vi "骰子比大小.vi"() -> ()   [LabVIEW 2014]
panel:
  in  "Listbox 3":i32[](listbox)
  in  "Listbox 2":i32[](listbox)
  in  "Listbox":i32[](listbox)
  in  "遊戲開始":bool
  out "賺取/賠掉金額總計":i32
  out "歷經輪數":i32
  out "此輪賺取/賠掉金額":i32
  out "賭金金額":i32
  in  "Cluster 12":T1={"Color Box 4"=16448250, "Boolean 5"=FALSE, "Boolean 11"=FALSE, "Boolean 12"=FALSE, "Boolean 13"=FALSE, "Boolean 14"=FALSE, "Boolean 15"=FALSE}
  in  "Cluster 11":T2={"Color Box"=16777215, "Boolean 4"=FALSE, "Boolean 5"=FALSE, "Boolean 6"=FALSE, "Boolean 7"=FALSE, "Boolean 8"=FALSE}
  in  "Cluster 10":T3={"Color Box 2"=16777215, "Boolean 3"=FALSE, "Boolean 4"=FALSE, "Boolean 6"=FALSE, "Boolean 5"=FALSE}
  in  "Cluster 9":T4={"Color Box 2"=16777215, "Boolean"=FALSE, "Boolean 3"=FALSE, "Boolean 2"=FALSE}
  in  "Cluster 8":T5={"Color Box"=16777215, "Boolean"=FALSE, "Boolean 2"=FALSE}
  in  "Cluster 7":T6={"Color Box"=16777215, "Boolean"=FALSE}
  in  "Cluster 6":T1={"Color Box 4"=16448250, "Boolean 5"=FALSE, "Boolean 11"=FALSE, "Boolean 12"=FALSE, "Boolean 13"=FALSE, "Boolean 14"=FALSE, "Boolean 15"=FALSE}
  in  "Cluster 5":T2={"Color Box"=16777215, "Boolean 4"=FALSE, "Boolean 5"=FALSE, "Boolean 6"=FALSE, "Boolean 7"=FALSE, "Boolean 8"=FALSE}
  in  "Cluster 4":T3={"Color Box 2"=16777215, "Boolean 3"=FALSE, "Boolean 4"=FALSE, "Boolean 6"=FALSE, "Boolean 5"=FALSE}
  in  "Cluster 3":T4={"Color Box 2"=16777215, "Boolean"=FALSE, "Boolean 3"=FALSE, "Boolean 2"=FALSE}
  in  "Cluster 2":T5={"Color Box"=16777215, "Boolean"=FALSE, "Boolean 2"=FALSE}
  in  "Cluster":T6={"Color Box"=16777215, "Boolean"=FALSE}
  in  "下注金額":i32=10 min=10 max=30
  in  "賠率":i32=1 min=1 max=5
  in  "進入下一輪":bool
  in  "停止擲骰子":bool
  in  "退出遊戲":bool
  out "莊家骰子點數":i32
  out "玩家骰子點數":i32
  # "遊戲介紹:"
  # "遊戲操作:"
  # "注意事項:"
  # "看完以上說明都沒問題的話，\n就可以按下遊戲開始開始遊玩囉!\n                         ↓"
  # "莊家骰子點數"
  # "玩家骰子點數"
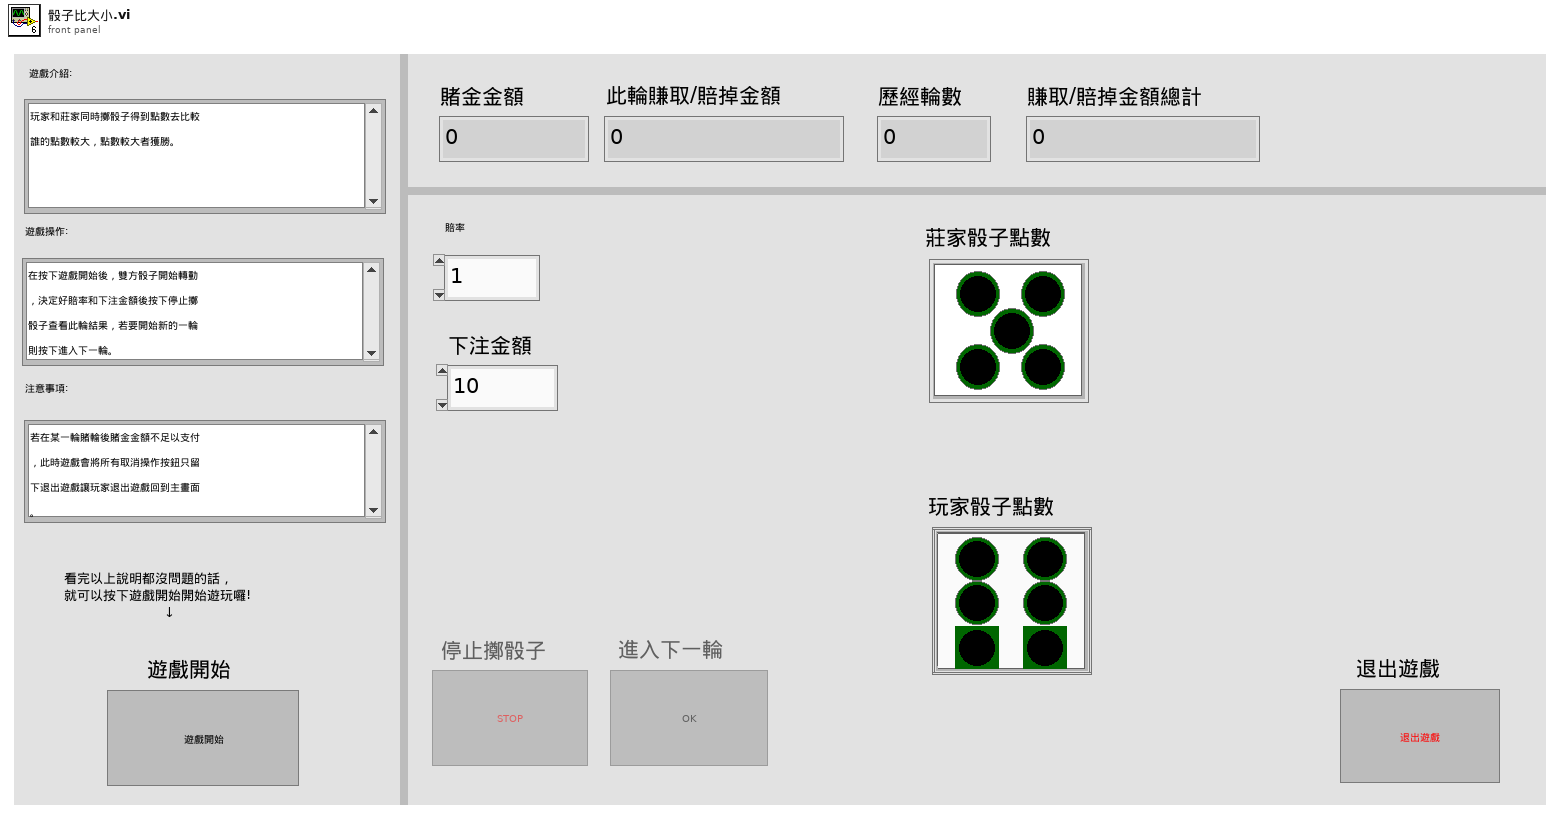
[diagram p1: front panel]
types:
  T1 = typedef "點數六.ctl" = cluster{"Color Box 4":u32, "Boolean 5":bool, "Boolean 11":bool, "Boolean 12":bool, "Boolean 13":bool, "Boolean 14":bool, "Boolean 15":bool}
  T2 = typedef "き.ctl" = cluster{"Color Box":u32, "Boolean 4":bool, "Boolean 5":bool, "Boolean 6":bool, "Boolean 7":bool, "Boolean 8":bool}
  T3 = typedef "點數四.ctl" = cluster{"Color Box 2":u32, "Boolean 3":bool, "Boolean 4":bool, "Boolean 6":bool, "Boolean 5":bool}
  T4 = typedef "點數三.ctl" = cluster{"Color Box 2":u32, "Boolean":bool, "Boolean 3":bool, "Boolean 2":bool}
  T5 = typedef "點數二.ctl" = cluster{"Color Box":u32, "Boolean":bool, "Boolean 2":bool}
  T6 = typedef "點數一.ctl" = cluster{"Color Box":u32, "Boolean":bool}
  T7 = enum16{"restart", "wait start button press", "compare", "throw dice", "init"}
  T8 = enum8{"Enabled", "Disabled", "Disabled and Grayed Out"}
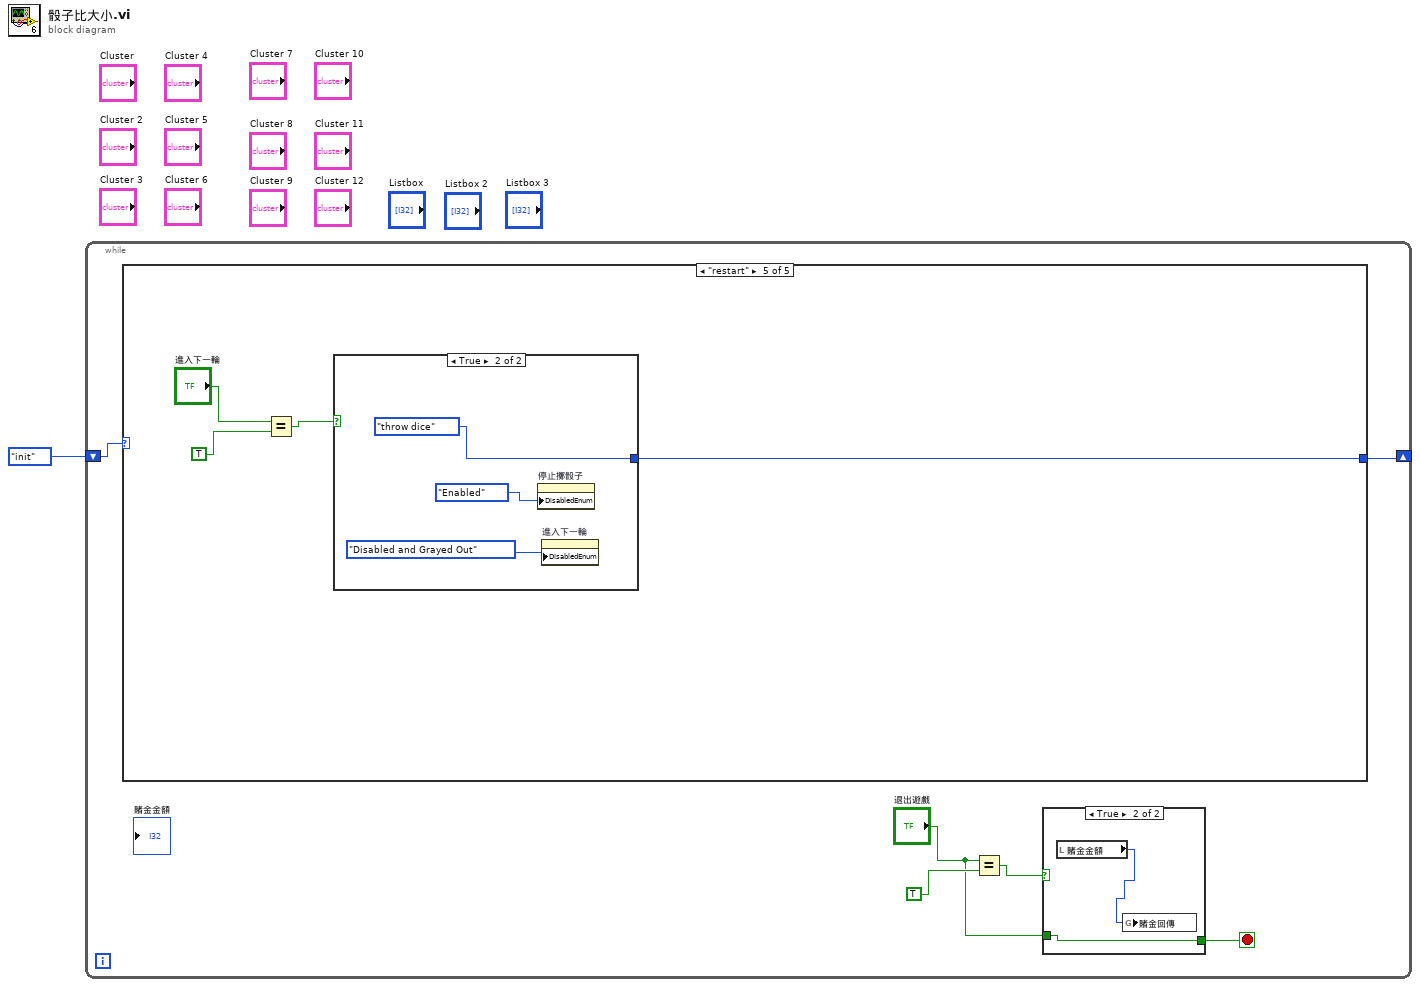
[diagram p0: block diagram]
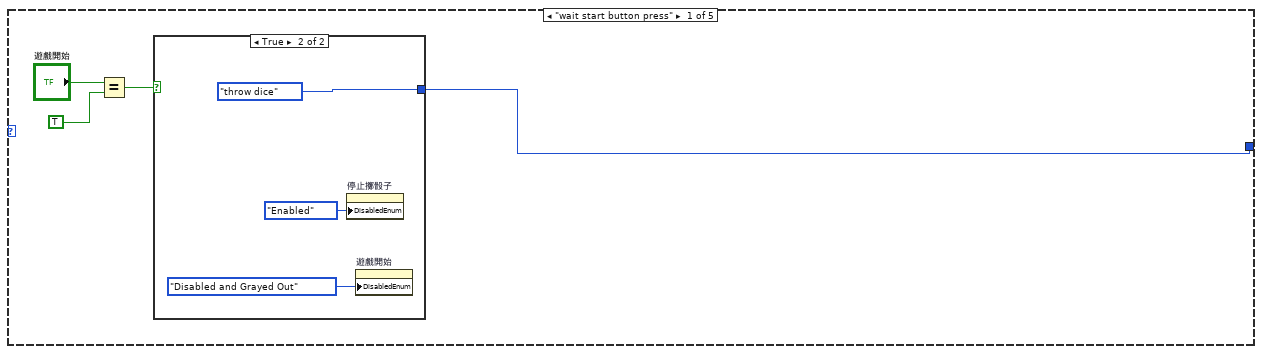
[diagram p3: hidden frame]
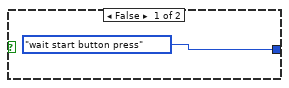
[diagram p4: hidden frame]
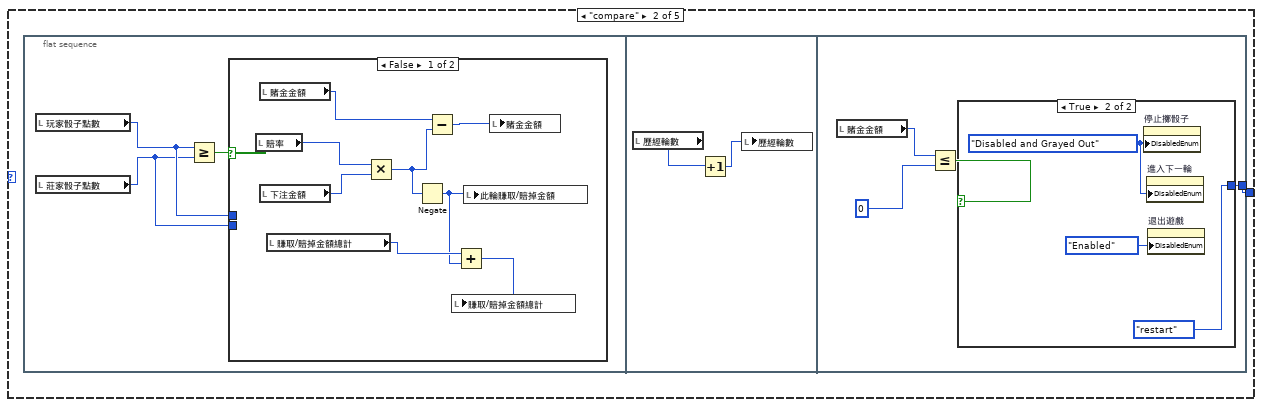
[diagram p5: hidden frame]
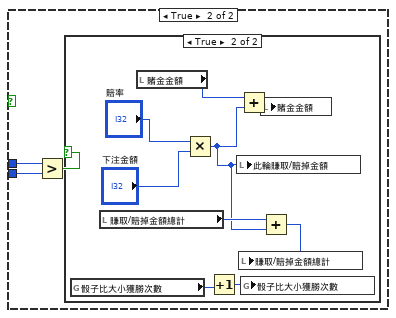
[diagram p6: hidden frame]
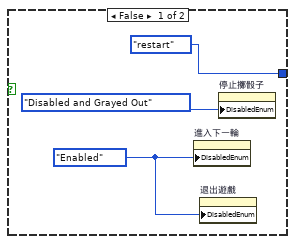
[diagram p8: hidden frame]
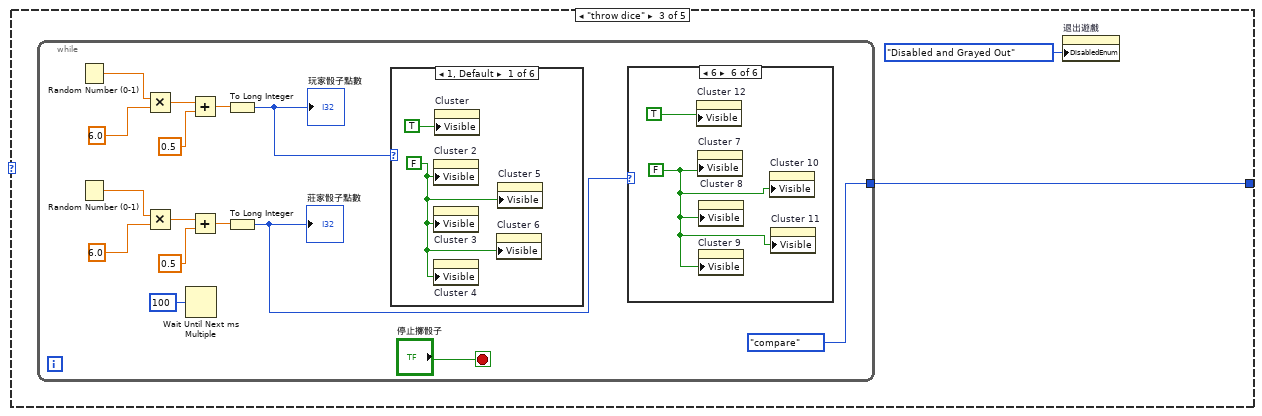
[diagram p9: hidden frame]
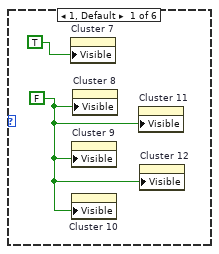
[diagram p10: hidden frame]
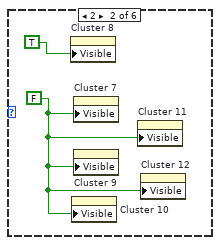
[diagram p11: hidden frame]
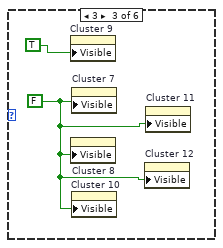
[diagram p12: hidden frame]
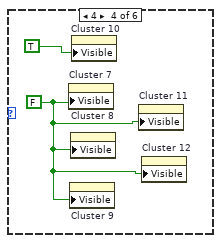
[diagram p13: hidden frame]
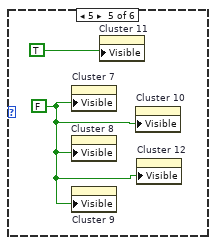
[diagram p14: hidden frame]
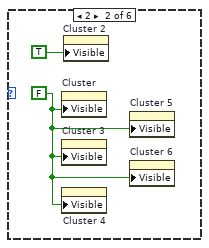
[diagram p15: hidden frame]
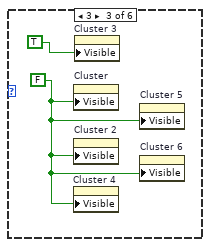
[diagram p16: hidden frame]
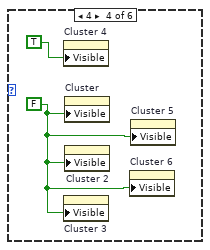
[diagram p17: hidden frame]
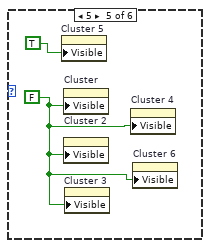
[diagram p18: hidden frame]
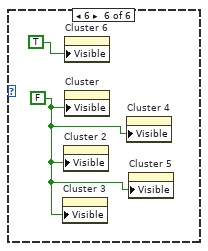
[diagram p19: hidden frame]
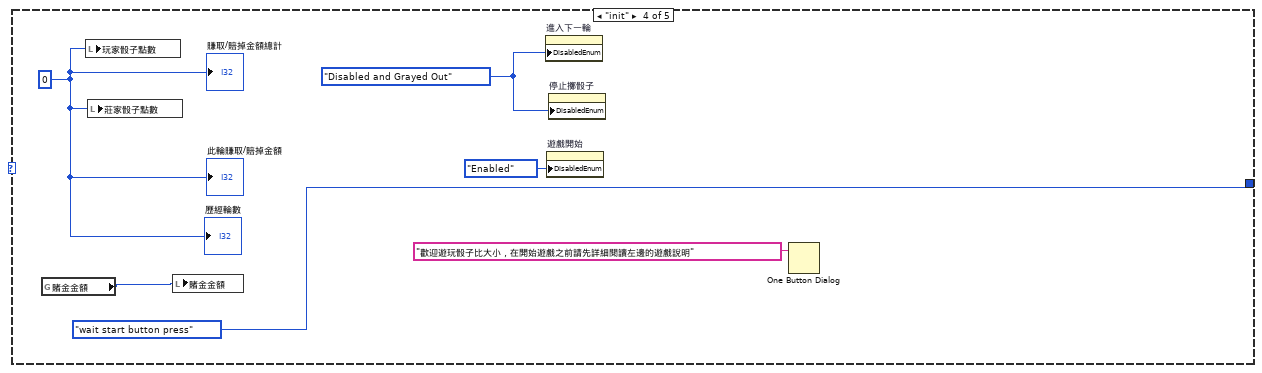
[diagram p20: hidden frame]
diagram:
  n1 = while {
    shift-right: [w6] -> _
    shift-left: T7."init" -> [w7]
    stop <- w3 stop-if-true
    n2 = case shown="\"restart\"" w7 {
      tunnel: [w11 w19 w56 T7."wait start button press" w102] -> w6
      frame "wait start button press" {
        n3 = Equal?(x="遊戲開始", y=TRUE) -> (x = y?=w12:bool)
        n4 = case shown="True" w12 {
          tunnel: [T7."wait start button press" T7."throw dice"] -> w11
          frame False {
          }
          frame True {
            n5 = property on="停止擲骰子" class="Bool"("DisabledEnum"=T8."Enabled" ("Disabled")) -> ()  [unwired: 2 in, 2 out]
            n6 = property on="遊戲開始" class="Bool (strict)"("DisabledEnum"=T8."Disabled and Grayed Out" ("Disabled")) -> ()  [unwired: 2 in, 2 out]
          }
        }
      }
      frame "compare" {
        n7 = flat-sequence {
          tunnel: [w45] -> w19
          frame #0 {
            n8 = local read "玩家骰子點數"() -> (w21:i32)
            n9 = local read "莊家骰子點數"() -> (w20:i32)
            n10 = Greater Or Equal?(x=w21, y=w20) -> (x >= y?=w22:bool)
            n11 = case shown="False" w22 {
              tunnel: w21 -> [_ w33]
              tunnel: w20 -> [_ w32]
              frame False {
                n12 = local read "賠率"() -> (w30:i32)
                n13 = local read "賭金金額"() -> (w28:i32)
                n14 = local read "下注金額"() -> (w29:i32)
                n15 = local read "賺取/賠掉金額總計"() -> (w25:i32)
                n16 = Multiply(x=w30, y=w29) -> (x*y=w26:i32)
                n17 = Negate(x=w26) -> (-x=w24:i32)
                n18 = Subtract(x=w28, y=w26) -> (x-y=w27:i32)
                n19 = Add(x=w25, y=w24) -> (x+y=w23:i32)
                n20 = local write "賺取/賠掉金額總計"(w23) -> ()
                n21 = local write "此輪賺取/賠掉金額"(w24) -> ()
                n22 = local write "賭金金額"(w27) -> ()
              }
              frame True {
                n23 = Greater?(x=w33, y=w32) -> (0:w31:bool)
                n24 = case shown="True" w31 {
                  frame False {
                  }
                  frame True {
                    n25 = global read "global variable-骰子比大小獲勝次數.vi" "骰子比大小獲勝次數"() -> (w34:i32)
                    n26 = local read "賺取/賠掉金額總計"() -> (w38:i32)
                    n27 = local read "賭金金額"() -> (w40:i32)
                    n28 = Multiply(x="賠率", y="下注金額") -> (x*y=w37:i32)
                    n29 = Increment(x=w34) -> (x+1=w35:i32)
                    n30 = local write "此輪賺取/賠掉金額"(w37) -> ()
                    n31 = Add(x=w40, y=w37) -> (x+y=w39:i32)
                    n32 = global write "global variable-骰子比大小獲勝次數.vi" "骰子比大小獲勝次數"(w35) -> ()
                    n33 = local write "賭金金額"(w39) -> ()
                    n34 = Add(x=w38, y=w37) -> (x+y=w36:i32)
                    n35 = local write "賺取/賠掉金額總計"(w36) -> ()
                  }
                }
              }
            }
          }
          frame #1 {
            n36 = local read "歷經輪數"() -> (w44:i32)
            n37 = Increment(x=w44) -> (x+1=w43:i32)
            n38 = local write "歷經輪數"(w43) -> ()
          }
          frame #2 {
            n39 = local read "賭金金額"() -> (w48:i32)
            n40 = Less Or Equal?(x=w48, y=0) -> (x <= y?=w46:bool)
            n41 = case shown="True" w46 {
              tunnel: [T7."restart" T7."restart"] -> w45
              frame False {
                w49 = T8."Enabled" ("Disabled")
                n42 = property on="進入下一輪" class="Bool"("DisabledEnum"=w49) -> ()  [unwired: 2 in, 2 out]
                n43 = property on="退出遊戲" class="Bool"("DisabledEnum"=w49) -> ()  [unwired: 2 in, 2 out]
                n44 = property on="停止擲骰子" class="Bool"("DisabledEnum"=T8."Disabled and Grayed Out" ("Disabled")) -> ()  [unwired: 2 in, 2 out]
              }
              frame True {
                w54 = T8."Disabled and Grayed Out" ("Disabled")
                n45 = property on="停止擲骰子" class="Bool"("DisabledEnum"=w54) -> ()  [unwired: 2 in, 2 out]
                n46 = property on="進入下一輪" class="Bool"("DisabledEnum"=w54) -> ()  [unwired: 2 in, 2 out]
                n47 = property on="退出遊戲" class="Bool"("DisabledEnum"=T8."Enabled" ("Disabled")) -> ()  [unwired: 2 in, 2 out]
              }
            }
          }
        }
      }
      frame "throw dice" {
        n48 = while {
          tunnel: [T7."compare"] -> w56
          stop <- "停止擲骰子" stop-if-true
          n49 = Random Number (0-1)() -> (number: 0 to 1=w71:dbl)
          n50 = Random Number (0-1)() -> (number: 0 to 1=w65:dbl)
          n51 = Multiply(x=w71, y=6.0) -> (x*y=w69:dbl)
          n52 = Multiply(x=w65, y=6.0) -> (x*y=w63:dbl)
          n53 = Wait Until Next ms Multiple(millisecond multiple=u32 100) -> ()  [unwired: 1 out]
          n54 = Add(x=w69, y=0.5) -> (x+y=w67:dbl)
          n55 = Add(x=w63, y=0.5) -> (x+y=w61:dbl)
          n56 = To Long Integer(number=w67) -> (32bit integer=w58:i32)
          "玩家骰子點數" <- w58
          n57 = To Long Integer(number=w61) -> (32bit integer=w57:i32)
          "莊家骰子點數" <- w57
          n58 = case shown="1, Default" w58 {
            frame 1, Default {
              w84 = FALSE
              n59 = property on="Cluster 2" class="Clust (strict)"("Visible"=w84) -> ()  [unwired: 2 in, 2 out]
              n60 = property on="Cluster 3" class="Clust (strict)"("Visible"=w84) -> ()  [unwired: 2 in, 2 out]
              n61 = property on="Cluster 4" class="Clust (strict)"("Visible"=w84) -> ()  [unwired: 2 in, 2 out]
              n62 = property on="Cluster" class="Clust (strict)"("Visible"=TRUE) -> ()  [unwired: 2 in, 2 out]
              n63 = property on="Cluster 6" class="Clust (strict)"("Visible"=w84) -> ()  [unwired: 2 in, 2 out]
              n64 = property on="Cluster 5" class="Clust (strict)"("Visible"=w84) -> ()  [unwired: 2 in, 2 out]
            }
            frame 2 {
              w86 = FALSE
              n65 = property on="Cluster" class="Clust (strict)"("Visible"=w86) -> ()  [unwired: 2 in, 2 out]
              n66 = property on="Cluster 3" class="Clust (strict)"("Visible"=w86) -> ()  [unwired: 2 in, 2 out]
              n67 = property on="Cluster 4" class="Clust (strict)"("Visible"=w86) -> ()  [unwired: 2 in, 2 out]
              n68 = property on="Cluster 2" class="Clust (strict)"("Visible"=TRUE) -> ()  [unwired: 2 in, 2 out]
              n69 = property on="Cluster 5" class="Clust (strict)"("Visible"=w86) -> ()  [unwired: 2 in, 2 out]
              n70 = property on="Cluster 6" class="Clust (strict)"("Visible"=w86) -> ()  [unwired: 2 in, 2 out]
            }
            frame 3 {
              w88 = FALSE
              n71 = property on="Cluster" class="Clust (strict)"("Visible"=w88) -> ()  [unwired: 2 in, 2 out]
              n72 = property on="Cluster 2" class="Clust (strict)"("Visible"=w88) -> ()  [unwired: 2 in, 2 out]
              n73 = property on="Cluster 4" class="Clust (strict)"("Visible"=w88) -> ()  [unwired: 2 in, 2 out]
              n74 = property on="Cluster 3" class="Clust (strict)"("Visible"=TRUE) -> ()  [unwired: 2 in, 2 out]
              n75 = property on="Cluster 5" class="Clust (strict)"("Visible"=w88) -> ()  [unwired: 2 in, 2 out]
              n76 = property on="Cluster 6" class="Clust (strict)"("Visible"=w88) -> ()  [unwired: 2 in, 2 out]
            }
            frame 4 {
              w90 = FALSE
              n77 = property on="Cluster 4" class="Clust (strict)"("Visible"=TRUE) -> ()  [unwired: 2 in, 2 out]
              n78 = property on="Cluster 3" class="Clust (strict)"("Visible"=w90) -> ()  [unwired: 2 in, 2 out]
              n79 = property on="Cluster" class="Clust (strict)"("Visible"=w90) -> ()  [unwired: 2 in, 2 out]
              n80 = property on="Cluster 2" class="Clust (strict)"("Visible"=w90) -> ()  [unwired: 2 in, 2 out]
              n81 = property on="Cluster 6" class="Clust (strict)"("Visible"=w90) -> ()  [unwired: 2 in, 2 out]
              n82 = property on="Cluster 5" class="Clust (strict)"("Visible"=w90) -> ()  [unwired: 2 in, 2 out]
            }
            frame 5 {
              w92 = FALSE
              n83 = property on="Cluster 5" class="Clust (strict)"("Visible"=TRUE) -> ()  [unwired: 2 in, 2 out]
              n84 = property on="Cluster" class="Clust (strict)"("Visible"=w92) -> ()  [unwired: 2 in, 2 out]
              n85 = property on="Cluster 2" class="Clust (strict)"("Visible"=w92) -> ()  [unwired: 2 in, 2 out]
              n86 = property on="Cluster 3" class="Clust (strict)"("Visible"=w92) -> ()  [unwired: 2 in, 2 out]
              n87 = property on="Cluster 4" class="Clust (strict)"("Visible"=w92) -> ()  [unwired: 2 in, 2 out]
              n88 = property on="Cluster 6" class="Clust (strict)"("Visible"=w92) -> ()  [unwired: 2 in, 2 out]
            }
            frame 6 {
              w94 = FALSE
              n89 = property on="Cluster 3" class="Clust (strict)"("Visible"=w94) -> ()  [unwired: 2 in, 2 out]
              n90 = property on="Cluster 2" class="Clust (strict)"("Visible"=w94) -> ()  [unwired: 2 in, 2 out]
              n91 = property on="Cluster 6" class="Clust (strict)"("Visible"=TRUE) -> ()  [unwired: 2 in, 2 out]
              n92 = property on="Cluster" class="Clust (strict)"("Visible"=w94) -> ()  [unwired: 2 in, 2 out]
              n93 = property on="Cluster 4" class="Clust (strict)"("Visible"=w94) -> ()  [unwired: 2 in, 2 out]
              n94 = property on="Cluster 5" class="Clust (strict)"("Visible"=w94) -> ()  [unwired: 2 in, 2 out]
            }
          }
          n95 = case shown="6" w57 {
            frame 1, Default {
              w72 = FALSE
              n96 = property on="Cluster 7" class="Clust (strict)"("Visible"=TRUE) -> ()  [unwired: 2 in, 2 out]
              n97 = property on="Cluster 9" class="Clust (strict)"("Visible"=w72) -> ()  [unwired: 2 in, 2 out]
              n98 = property on="Cluster 10" class="Clust (strict)"("Visible"=w72) -> ()  [unwired: 2 in, 2 out]
              n99 = property on="Cluster 8" class="Clust (strict)"("Visible"=w72) -> ()  [unwired: 2 in, 2 out]
              n100 = property on="Cluster 11" class="Clust (strict)"("Visible"=w72) -> ()  [unwired: 2 in, 2 out]
              n101 = property on="Cluster 12" class="Clust (strict)"("Visible"=w72) -> ()  [unwired: 2 in, 2 out]
            }
            frame 2 {
              w74 = FALSE
              n102 = property on="Cluster 8" class="Clust (strict)"("Visible"=TRUE) -> ()  [unwired: 2 in, 2 out]
              n103 = property on="Cluster 10" class="Clust (strict)"("Visible"=w74) -> ()  [unwired: 2 in, 2 out]
              n104 = property on="Cluster 7" class="Clust (strict)"("Visible"=w74) -> ()  [unwired: 2 in, 2 out]
              n105 = property on="Cluster 9" class="Clust (strict)"("Visible"=w74) -> ()  [unwired: 2 in, 2 out]
              n106 = property on="Cluster 11" class="Clust (strict)"("Visible"=w74) -> ()  [unwired: 2 in, 2 out]
              n107 = property on="Cluster 12" class="Clust (strict)"("Visible"=w74) -> ()  [unwired: 2 in, 2 out]
            }
            frame 3 {
              w76 = FALSE
              n108 = property on="Cluster 9" class="Clust (strict)"("Visible"=TRUE) -> ()  [unwired: 2 in, 2 out]
              n109 = property on="Cluster 8" class="Clust (strict)"("Visible"=w76) -> ()  [unwired: 2 in, 2 out]
              n110 = property on="Cluster 7" class="Clust (strict)"("Visible"=w76) -> ()  [unwired: 2 in, 2 out]
              n111 = property on="Cluster 10" class="Clust (strict)"("Visible"=w76) -> ()  [unwired: 2 in, 2 out]
              n112 = property on="Cluster 12" class="Clust (strict)"("Visible"=w76) -> ()  [unwired: 2 in, 2 out]
              n113 = property on="Cluster 11" class="Clust (strict)"("Visible"=w76) -> ()  [unwired: 2 in, 2 out]
            }
            frame 4 {
              w78 = FALSE
              n114 = property on="Cluster 7" class="Clust (strict)"("Visible"=w78) -> ()  [unwired: 2 in, 2 out]
              n115 = property on="Cluster 9" class="Clust (strict)"("Visible"=w78) -> ()  [unwired: 2 in, 2 out]
              n116 = property on="Cluster 8" class="Clust (strict)"("Visible"=w78) -> ()  [unwired: 2 in, 2 out]
              n117 = property on="Cluster 10" class="Clust (strict)"("Visible"=TRUE) -> ()  [unwired: 2 in, 2 out]
              n118 = property on="Cluster 11" class="Clust (strict)"("Visible"=w78) -> ()  [unwired: 2 in, 2 out]
              n119 = property on="Cluster 12" class="Clust (strict)"("Visible"=w78) -> ()  [unwired: 2 in, 2 out]
            }
            frame 5 {
              w80 = FALSE
              n120 = property on="Cluster 7" class="Clust (strict)"("Visible"=w80) -> ()  [unwired: 2 in, 2 out]
              n121 = property on="Cluster 8" class="Clust (strict)"("Visible"=w80) -> ()  [unwired: 2 in, 2 out]
              n122 = property on="Cluster 9" class="Clust (strict)"("Visible"=w80) -> ()  [unwired: 2 in, 2 out]
              n123 = property on="Cluster 11" class="Clust (strict)"("Visible"=TRUE) -> ()  [unwired: 2 in, 2 out]
              n124 = property on="Cluster 10" class="Clust (strict)"("Visible"=w80) -> ()  [unwired: 2 in, 2 out]
              n125 = property on="Cluster 12" class="Clust (strict)"("Visible"=w80) -> ()  [unwired: 2 in, 2 out]
            }
            frame 6 {
              w82 = FALSE
              n126 = property on="Cluster 12" class="Clust (strict)"("Visible"=TRUE) -> ()  [unwired: 2 in, 2 out]
              n127 = property on="Cluster 7" class="Clust (strict)"("Visible"=w82) -> ()  [unwired: 2 in, 2 out]
              n128 = property on="Cluster 8" class="Clust (strict)"("Visible"=w82) -> ()  [unwired: 2 in, 2 out]
              n129 = property on="Cluster 9" class="Clust (strict)"("Visible"=w82) -> ()  [unwired: 2 in, 2 out]
              n130 = property on="Cluster 10" class="Clust (strict)"("Visible"=w82) -> ()  [unwired: 2 in, 2 out]
              n131 = property on="Cluster 11" class="Clust (strict)"("Visible"=w82) -> ()  [unwired: 2 in, 2 out]
            }
          }
        }
        n132 = property on="退出遊戲" class="Bool"("DisabledEnum"=T8."Disabled and Grayed Out" ("Disabled")) -> ()  [unwired: 2 in, 2 out]
      }
      frame "init" {
        w98 = T8."Disabled and Grayed Out" ("Disabled")
        w100 = 0
        n133 = global read "global variable-賭金金額.vi" "賭金金額"() -> (w97:i32)
        n134 = local write "玩家骰子點數"(w100) -> ()
        n135 = local write "莊家骰子點數"(w100) -> ()
        n136 = local write "賭金金額"(w97) -> ()
        n137 = property on="進入下一輪" class="Bool"("DisabledEnum"=w98) -> ()  [unwired: 2 in, 2 out]
        n138 = property on="遊戲開始" class="Bool (strict)"("DisabledEnum"=T8."Enabled" ("Disabled")) -> ()  [unwired: 2 in, 2 out]
        n139 = property on="停止擲骰子" class="Bool"("DisabledEnum"=w98) -> ()  [unwired: 2 in, 2 out]
        n140 = One Button Dialog(message="歡迎遊玩骰子比大小，在開始遊戲之前請先詳細閱讀左邊的遊戲說明") -> ()  [unwired: 1 in, 1 out]
        "此輪賺取/賠掉金額" <- w100
        "歷經輪數" <- w100
        "賺取/賠掉金額總計" <- w100
      }
      frame "restart" {
        n141 = Equal?(x="進入下一輪", y=TRUE) -> (x = y?=w103:bool)
        n142 = case shown="True" w103 {
          tunnel: [T7."restart" T7."throw dice"] -> w102
          frame False {
          }
          frame True {
            n143 = property on="停止擲骰子" class="Bool"("DisabledEnum"=T8."Enabled" ("Disabled")) -> ()  [unwired: 2 in, 2 out]
            n144 = property on="進入下一輪" class="Bool"("DisabledEnum"=T8."Disabled and Grayed Out" ("Disabled")) -> ()  [unwired: 2 in, 2 out]
          }
        }
      }
    }
    n145 = Equal?(x="退出遊戲", y=TRUE) -> (x = y?=w4:bool)
    n146 = case shown="True" w4 {
      tunnel: "退出遊戲" -> [w8 w10]
      tunnel: [w8 w10] -> w3
      frame False {
      }
      frame True {
        n147 = local read "賭金金額"() -> (w9:i32)
        n148 = global write "global variable-賭金回傳.vi" "賭金回傳"(w9) -> ()
      }
    }
  }
